vi "send_false_case.vi"(8 "error in (no error)":errorcluster, 11 "queue in":refnum<queue>) -> (0 "error out":errorcluster, 2 "message":string, 3 "error?":bool)   [LabVIEW 2015]
uses:
  <vilib>/Utility/error.llb/DialogType.ctl
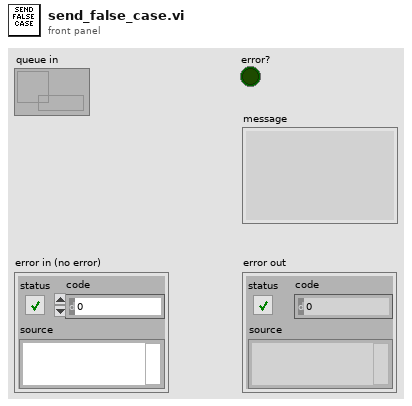
[diagram p1: front panel]
types:
  T1 = typedef "DialogType.ctl" = u16
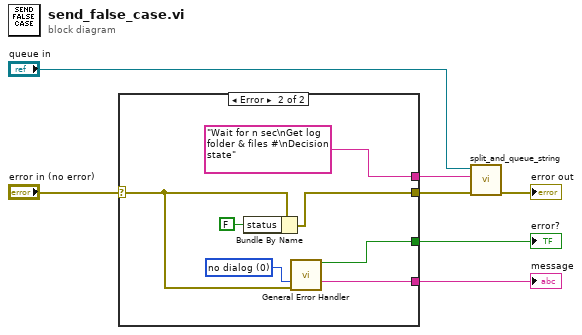
[diagram p0: block diagram]
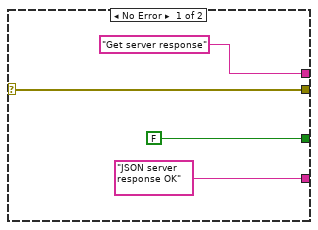
[diagram p2: hidden frame]
diagram:
  n1 = case shown="Error" "error in (no error)" {
    selector: "error in (no error)" -> [w11 w14]
    tunnel: [w11 w18] -> w5
    tunnel: ["Get server response" "Wait for n sec\nGet log folder & files #\nDecision state"] -> w4
    tunnel: ["JSON server response OK" w16] -> w6
    tunnel: [FALSE w15] -> w7
    frame No Error {
    }
    frame Error {
      w12 = T1 0 items=["no dialog", "OK message", "continue or stop message", "OK message + warnings", "continue/stop + warnings"] ("type of dialog (OK msg:1)")
      n2 = Bundle By Name(cluster=w14, "status"=FALSE) -> (w18:errorcluster)
      n3 = call <vilib>:"General Error Handler.vi"("type of dialog (OK msg:1)"=w12, "error in (no error)"=w14) -> ("error?"=w15:bool, "message"=w16:string)  [unwired: 9 in, 3 out]
    }
  }
  "error?" <- w7
  "message" <- w6
  n4 = call "split_and_queue_string.vi"("error in (no error)"=w5, "program string"=w4, "queue in"="queue in") -> ("error out"=→"error out":errorcluster)  [unwired: 7 in, 1 out]
